vi "GetVIActivationEvent.vi"(8 "error in (no error)":errorcluster, 11 "VI Activation in":refnum<class "VIActivation.lvclass">) -> (0 "error out":errorcluster, 2 "VIActivation":refnum<user-event>, 3 "VI Activation out":refnum<class "VIActivation.lvclass">)   [LabVIEW 2021, in "VIActivation.lvlib" / "VIActivation.lvclass"]
uses:
  VIActivation.lvclass
  VIActivation.lvclass/VIActivation.ctl
  VIActivationEvents.ctl
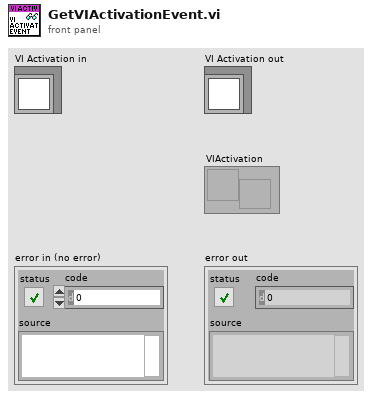
[diagram p1: front panel]
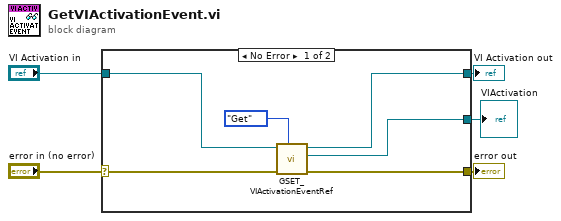
[diagram p0: block diagram]
diagram:
  n1 = case shown="No Error" "error in (no error)" {
    selector: "error in (no error)" -> [w11 w12]
    tunnel: [w10 _] -> w1
    tunnel: "VI Activation in" -> [w8 w13]
    tunnel: [w6 w12] -> w4
    tunnel: [w7 w13] -> w2
    frame No Error {
      n2 = call "GSET_VIActivationEventRef.vi"("Action"=enum16{"Get", "Set"}."Get", "error in (no error)"=w11, "Menu in"=w8) -> ("error out"=w6:errorcluster, "VIActivationEvent out"=w10:refnum<user-event>, "Menu out"=w7:refnum<class "VIActivation.lvclass">)  [unwired: 6 in]
    }
    frame Error {
    }
  }
  "VI Activation out" <- w2
  "error out" <- w4
  "VIActivation" <- w1
